vi "Get Source Node RTDestination.vi"(8 "error in (no error)":errorcluster, 11 "Node ref in":refnum<k20>) -> (0 "error out":errorcluster, 1 "Found ?":bool, 2 "RT Destination Node":refnum<k20>, 3 "Node ref out":refnum<k20>)   [LabVIEW 2018, in ".LVLIBP CD XML Updater.lvlib" / "Project XML Editor.lvclass"]
uses:
  Project XML Editor.lvclass
  <vilib>/xml/NI_XML.lvlib
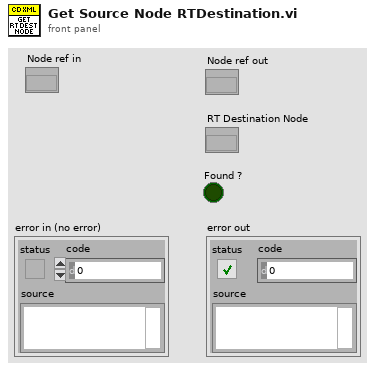
[diagram p1: front panel]
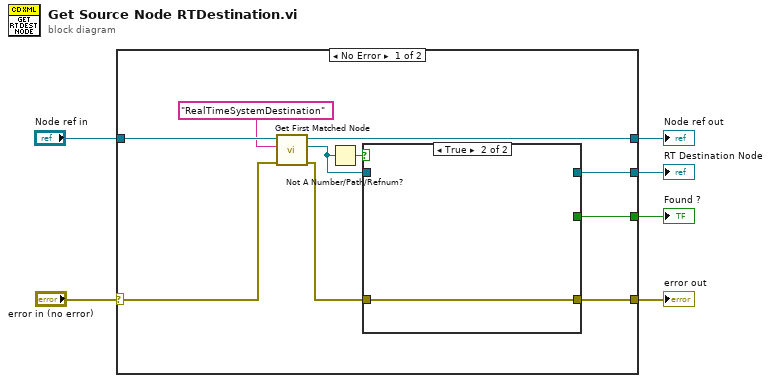
[diagram p0: block diagram]
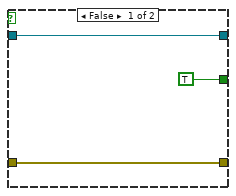
[diagram p2: hidden frame]
diagram:
  n1 = case shown="No Error" "error in (no error)" {
    selector: "error in (no error)" -> [w13 w22]
    tunnel: "Node ref in" -> [w15 w21]
    tunnel: [w12 w22] -> w4
    tunnel: [w11 w21] -> w3
    tunnel: [w8 _] -> w2
    tunnel: [w7 _] -> w1
    frame No Error {
      n2 = call <vilib>:"Get First Matched Node.vi"("error in (no error)"=w13, "XPath expression"="RealTimeSystemDestination", "node in"=w15) -> ("error out"=w16:errorcluster, "node result"=w10:refnum<k20>, "node out"=w11:refnum<k20>)  [unwired: 6 in]
      n3 = Not A Number/Path/Refnum?(number/path/refnum=w10) -> (NaN/Path/Refnum?=w9:bool)
      n4 = case shown="True" w9 {
        tunnel: w16 -> [w17 w20]
        tunnel: [w17 w20] -> w12
        tunnel: w10 -> [w18 _]
        tunnel: [TRUE _] -> w8
        tunnel: [w18 _] -> w7
        frame False {
        }
        frame True {
        }
      }
    }
    frame Error {
    }
  }
  "error out" <- w4
  "Node ref out" <- w3
  "Found ?" <- w2
  "RT Destination Node" <- w1
